vi "UpdateStatusPub.vi"(8 "error in (no error)":errorcluster, 11 "S4GUI in":refnum<class "S4GUI.lvclass">) -> (0 "error out":errorcluster, 2 "STATUS cluster":T1, 3 "S4GUI out":refnum<class "S4GUI.lvclass">)   [LabVIEW 2018, in "S4GUI.lvclass"]
uses:
  S4GUI.lvclass
  S4GUI.lvclass/S4GUI.ctl
  Server/Server.lvclass/Server.ctl
  Acquisition/Acquisition.lvclass
  C:/Users/devstaff/sparc4/s4gui/Versao ZeroMQ REQ-REP/SPARC4_GUI -v1.0.0/Server/Server.lvclass
  Publisher/Publisher.lvclass
  Instrument/Instrument.lvclass
  Server/Server.lvclass
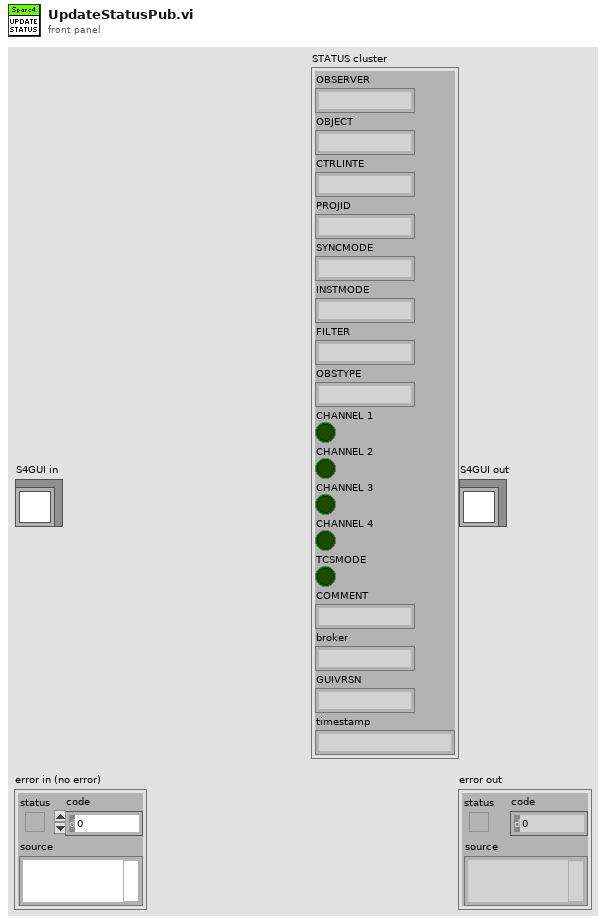
[diagram p1: front panel]
types:
  T1 = cluster{"OBSERVER":string, "OBJECT":string, "CTRLINTE":string, "PROJID":string, "SYNCMODE":string, "INSTMODE":string, "FILTER":string, "OBSTYPE":string, "CHANNEL 1":bool, "CHANNEL 2":bool, "CHANNEL 3":bool, "CHANNEL 4":bool, "TCSMODE":bool, "COMMENT":string, "broker":string, "GUIVRSN":string, "timestamp":string}
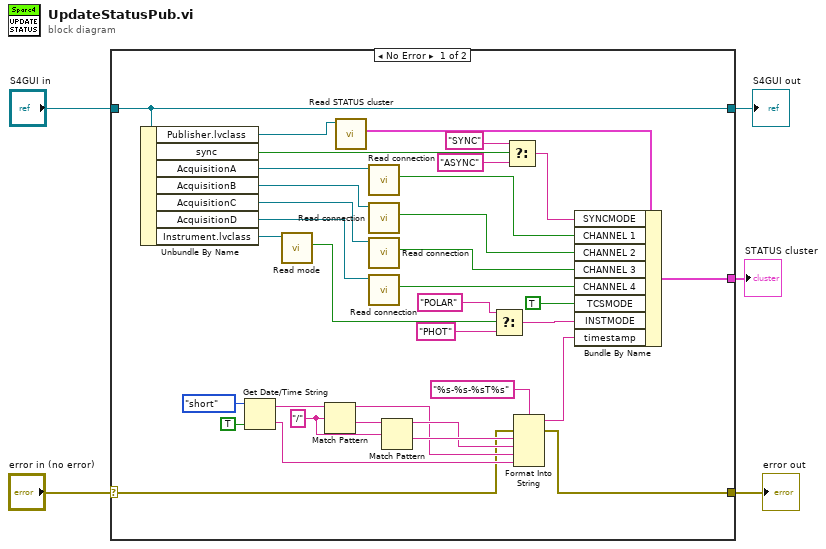
[diagram p0: block diagram]
diagram:
  n1 = case shown="No Error" "error in (no error)" {
    selector: "error in (no error)" -> [w7 w42]
    tunnel: [w6 w42] -> w4
    tunnel: [w39 w41] -> w2
    tunnel: "S4GUI in" -> [w39 w41]
    tunnel: [w40 _] -> w1
    frame No Error {
      w14 = "/" ("regular expression")
      n2 = Unbundle By Name(w39) -> ("Publisher.lvclass"=w22:refnum<class "Publisher.lvclass">, "sync"=w38:bool, "AcquisitionA"=w33:refnum<class "Acquisition.lvclass">, "AcquisitionB"=w31:refnum<class "Acquisition.lvclass">, "AcquisitionC"=w29:refnum<class "Acquisition.lvclass">, "AcquisitionD"=w27:refnum<class "Acquisition.lvclass">, "Instrument.lvclass"=w25:refnum<class "Instrument.lvclass">)
      n3 = Get Date/Time String(date format (0)=enum16{"short", "long", "abbreviated"}."short", want seconds? (F)=TRUE) -> (date string=w15:string, time string=w9:string)  [unwired: 1 in]
      n4 = call-dynamic "Read mode.vi"("Instrument in"=w25) -> ("mode"=w24:bool)  [unwired: 8 in, 2 out]
      n5 = Match Pattern(string=w15, regular expression=w14) -> (before substring=w10:string, after substring=w16:string)  [unwired: 1 in, 2 out]
      n6 = call-dynamic "Read STATUS cluster.vi"("Publisher in"=w22) -> ("STATUS cluster"=w21:T1)  [unwired: 8 in, 2 out]
      n7 = call "Read connection.vi"("Server in"=w33) -> ("connection"=w32:bool)  [unwired: 8 in, 2 out]
      n8 = call "Read connection.vi"("Server in"=w31) -> ("connection"=w30:bool)  [unwired: 8 in, 2 out]
      n9 = call "Read connection.vi"("Server in"=w29) -> ("connection"=w28:bool)  [unwired: 8 in, 2 out]
      n10 = call "Read connection.vi"("Server in"=w27) -> ("connection"=w26:bool)  [unwired: 8 in, 2 out]
      n11 = Match Pattern(string=w16, regular expression=w14) -> (before substring=w11:string, after substring=w12:string)  [unwired: 1 in, 2 out]
      n12 = Select(t="POLAR", s=w24, f="PHOT") -> (s? t:f=w23:string)
      n13 = Select(t="SYNC", s=w38, f="ASYNC") -> (s? t:f=w35:string)
      n14 = Format Into String(format string="%s-%s-%sT%s", error in=w7, w12, w11, w10, w9) -> (resulting string=w8:string, error out=w6:errorcluster)  [unwired: 1 in]
      n15 = Bundle By Name(cluster=w21, "SYNCMODE"=w35, "CHANNEL 1"=w32, "CHANNEL 2"=w30, "CHANNEL 3"=w28, "CHANNEL 4"=w26, "TCSMODE"=TRUE ("tcsmode"), "INSTMODE"=w23, "timestamp"=w8) -> (w40:T1)
    }
    frame Error {
    }
  }
  "error out" <- w4
  "S4GUI out" <- w2
  "STATUS cluster" <- w1
